vi "Read Measurement (Harmonics).vi"(6 "Timeout (10000 ms)":i32=10000 min=1, 8 "error in (no error)":errorcluster, 9 "Number of Item (15)":i32=15 min=1 max=64, 10 "Measure Item (1: Plural)":i32(ring)=1 items=["One", "Plural"], 11 "VISA resource name":refnum<visa-resource-name>) -> (0 "error out":errorcluster, 1 "Measurement":dbl[][](array[numeric]), 2 "Function":string[](array[string]), 3 "VISA resource name out":refnum<visa-resource-name>)   [LabVIEW 2021, in "Yokogawa WT1800 Series.lvlib"]
doc: "Queries the harmonic measurement numeric list data."
uses:
  <instrlib>/Yokogawa WT1800 Series/Yokogawa WT1800 Series.lvlib
  <instrlib>/Yokogawa WT1800 Series/Public/Data/Low Level/Fetch Measurement (Harmonics).vi
panel:
  # "Total        DC            1             2              3             4"
  # "ms"
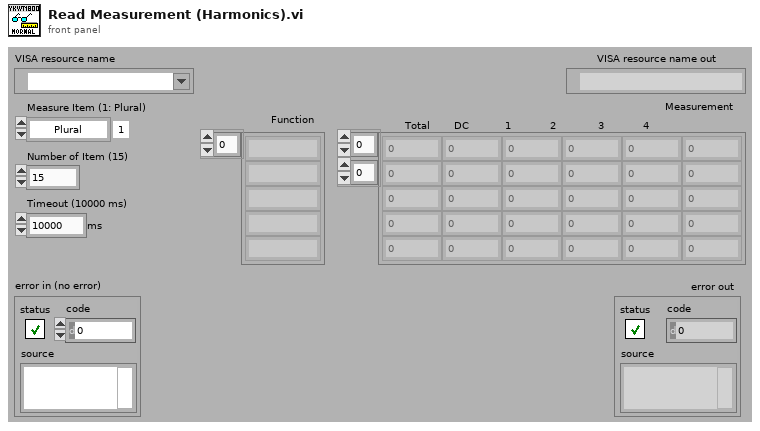
[diagram p1: front panel]
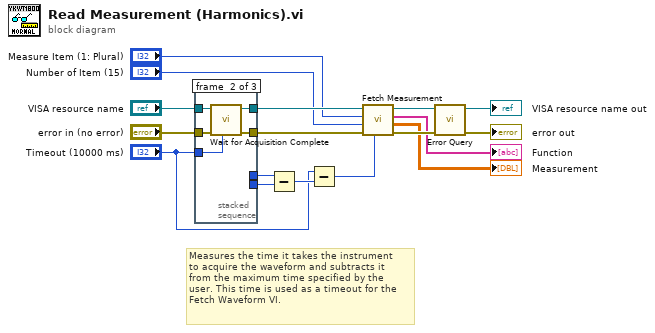
[diagram p0: block diagram]
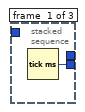
[diagram p2: hidden frame]
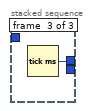
[diagram p3: hidden frame]
diagram:
  # "Measures the time it takes the instrument \nto acquire the waveform and subtracts it \nfrom the maximum time specified by the \nuser. This time is used as a timeout for the \nFetch Waveform VI."
  n1 = stacked-sequence {
    tunnel: "VISA resource name" -> [_ w22 _]
    tunnel: [_ w20 _] -> w16
    tunnel: "error in (no error)" -> [_ w21 _]
    tunnel: [_ w19 _] -> w17
    tunnel: [w18 _ _] -> w14
    tunnel: "Timeout (10000 ms)" -> [_ w23 _]
    tunnel: [_ _ w24] -> w15
    frame #0 {
      n2 = Tick Count (ms)() -> (millisecond timer value=w18:u32)
    }
    frame #1 {
      n3 = call <instrlib>:"Wait for Acquisition Complete.vi"("Timeout (10000 ms)"=w23, "error in (no error)"=w21, "VISA resource name"=w22) -> ("error out"=w19:errorcluster, "VISA resource name out"=w20:refnum<visa-resource-name>)  [unwired: 7 in]
    }
    frame #2 {
      n4 = Tick Count (ms)() -> (millisecond timer value=w24:u32)
    }
  }
  n5 = Subtract(x=w15, y=w14) -> (x-y=w12:u32)
  n6 = Subtract(x="Timeout (10000 ms)", y=w12) -> (x-y=w13:u32)
  n7 = call-poly <instrlib>:"Fetch Measurement.vi"("Timeout (10000 ms)"=w13, "error in (no error)"=w17, "Number of Item (15)"="Number of Item (15)", "Measure Item (1: Plural)"="Measure Item (1: Plural)", "VISA resource name"=w16) -> ("error out"=w11:errorcluster, "Measurement"=→"Measurement":dbl[][], "Function"=→"Function":string[], "VISA resource name out"=w10:refnum<visa-resource-name>)  [unwired: 3 in]
  n8 = call <instrlib>:"Error Query.vi"("error in (no error)"=w11, "VISA resource name"=w10) -> ("error out"=→"error out":errorcluster, "VISA resource name out"=→"VISA resource name out":refnum<visa-resource-name>)  [unwired: 6 in, 2 out]
